vi "ArrayMean.vi"(9 "Array":dbl[](array[numeric])) -> (1 "Mean":dbl)   [LabVIEW 2016]
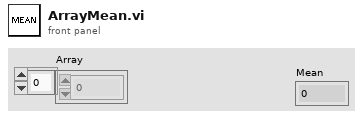
[diagram p1: front panel]
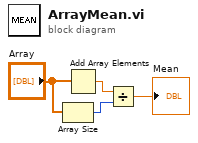
[diagram p0: block diagram]
diagram:
  n1 = Array Size(array="Array") -> (size(s)=w3:i32)
  n2 = Add Array Elements(numeric array="Array") -> (sum=w2:dbl)
  n3 = Divide(x=w2, y=w3) -> (x/y=→"Mean":dbl)
